vi "DAQMan Clear Specific Error.vi"(8 "error in":errorcluster, 11 "code":i32) -> (0 "error out":errorcluster)   [LabVIEW 2012]
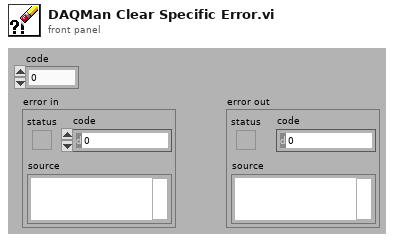
[diagram p1: front panel]
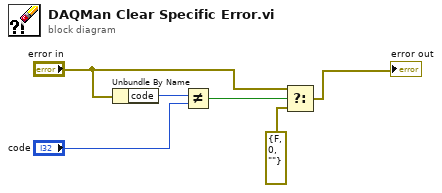
[diagram p0: block diagram]
diagram:
  n1 = Unbundle By Name("error in") -> ("code"=w1:i32)
  n2 = Not Equal?(x=w1, y="code") -> (x != y?=w3:bool)
  n3 = Select(t="error in", s=w3, f=errorcluster {"status"=FALSE, "code"=0, "source"=""}) -> (s? t:f=→"error out":errorcluster)
